vi "ASYNC_Adam_server.vi"(3 "Values":dbl[](array[numeric]) format="%.2f", 4 "Client Name":string="G3_3 HD", 5 "Channel Names":string[](array[string])) -> (0 "Scan Comments":string[](array[string]), 2 "Calibrated Units":dbl[](array[numeric]) format="%.2f")   [LabVIEW 2021]
uses:
  ADAM Client/Sub VIs/ADAM Controls/Channel_State.ctl
  ADAM Client/Sub VIs/ADAM Controls/Update_scan_value.ctl
  0eb1e5d3-c67c-5f4b-9ec6-5088df587a31.vi
  Anemometry/Anemometry Sub Vis/Globals/Preference_global.vi
panel:
  out "iteration":i32
  in  "delayBetweenADAMi/o(ms)":u32
  in  "Channel Name to Watch":string
  out "Call Chain":string[](array[string])
  # "Enter the Channel name that you want to watch"
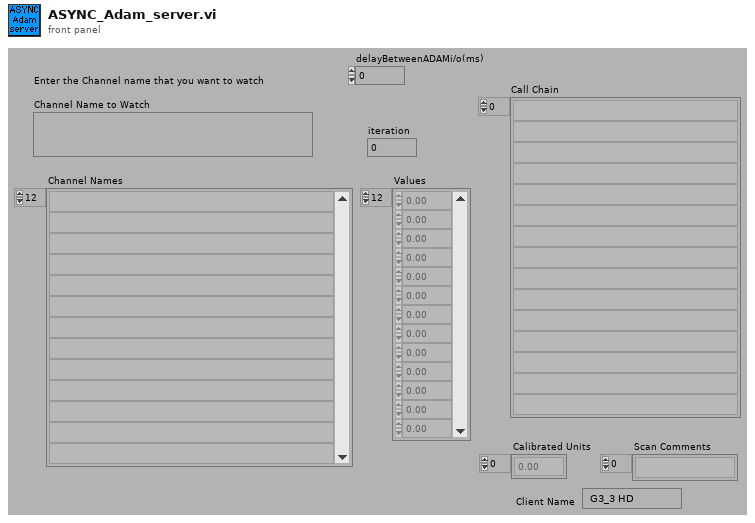
[diagram p1: front panel]
types:
  T1 = typedef "Channel_State.ctl" = enum16{"On", "Off", "Always On", "Always Off"}
  T2 = enum16{"Append to Global", "Read Global then Clear"}
  T3 = typedef "Update_scan_value.ctl" = cluster{"Channel Name":string, "New Value":dbl, "!Auto_Off":bool}
  T4 = typedef "Ch_description_ADAM.ctl" = cluster{"Ch Name":string, "Type":T5, "Function":T6, "Ch State":T1, "Calibration type":T7, "A":dbl, "B":dbl, "C":dbl, "D":dbl, "Comments":string, "Address":T8, "String":string, "Duty":u16}
  T5 = typedef "Module_type_ADAM.ctl" = string
  T6 = typedef "Function_ADAM.ctl" = enum16{"Analogue Input", "Digital Input", "Event counter", "Event rate", "Analogue Output", "Digital Output", "Relay Output"}
  T7 = typedef "Calib_type_ADAM.ctl" = string
  T8 = typedef "Address.ctl" = cluster{"Main":i32, "Ch.":i32, "Sub":i32, "Port Name":string}
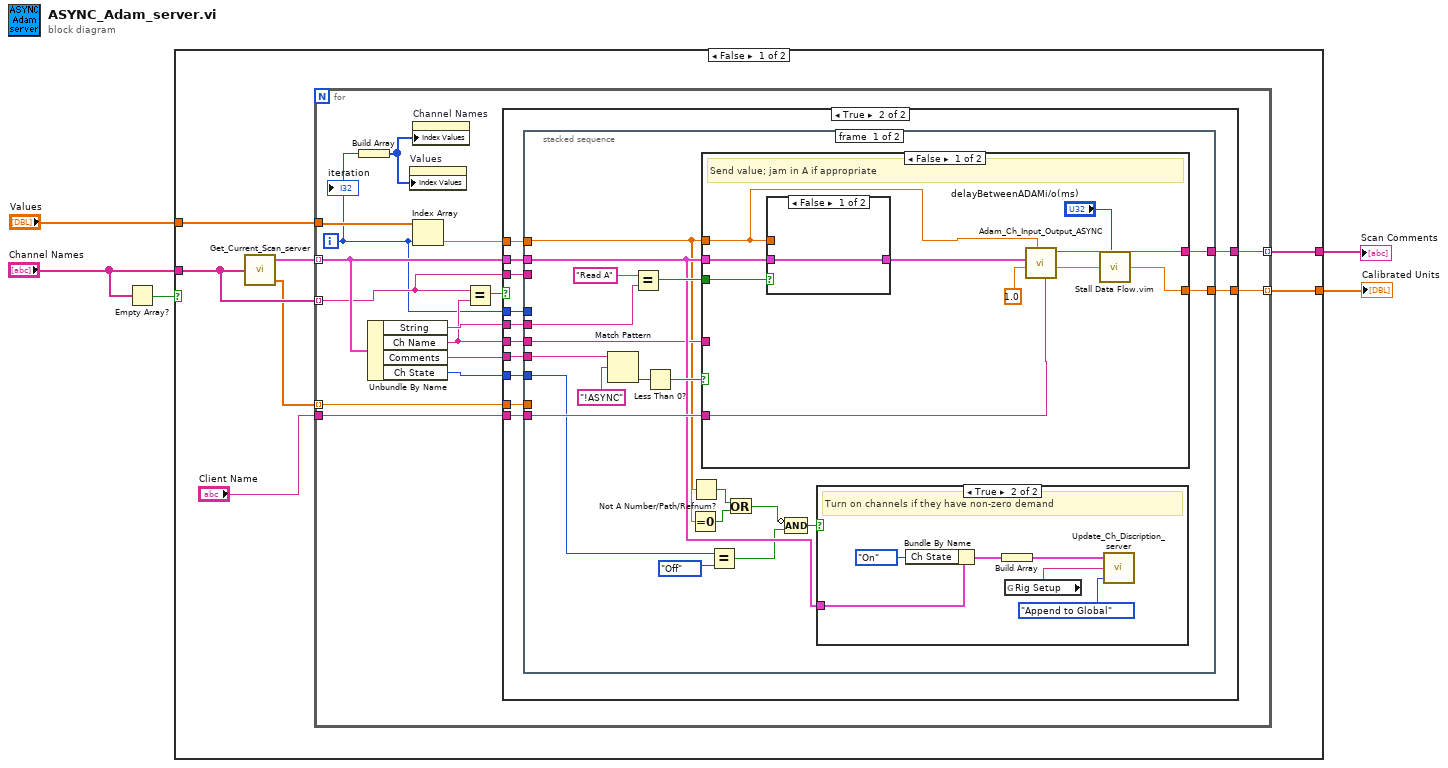
[diagram p0: block diagram]
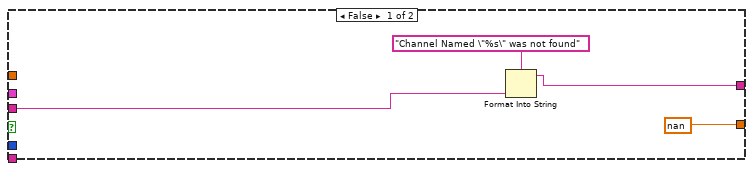
[diagram p2: hidden frame]
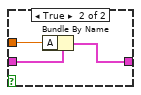
[diagram p4: hidden frame]
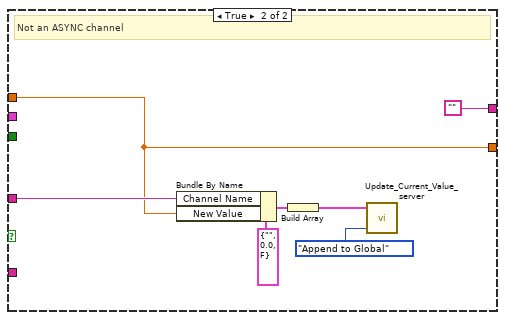
[diagram p5: hidden frame]
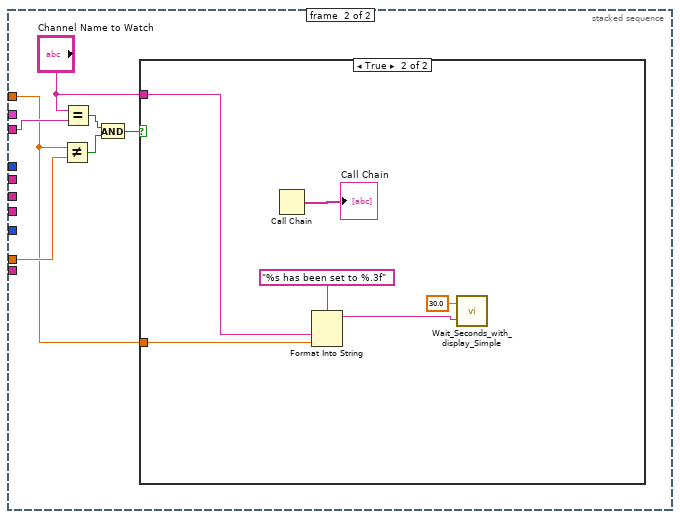
[diagram p6: hidden frame]
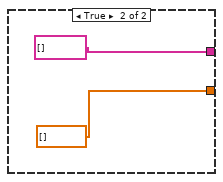
[diagram p8: hidden frame]
diagram:
  n1 = Empty Array?(array="Channel Names") -> (empty?=w3:bool)
  n2 = case shown="False" w3 {
    tunnel: "Channel Names" -> [w8 _]
    tunnel: [w10 dbl[] []] -> w5
    tunnel: [w9 string[] []] -> w4
    tunnel: "Values" -> [w7 _]
    frame False {
      n3 = call "Get_Current_Scan_server.vi"("Desired Channels"=w8) -> ("Ch Description Array"=w12:T4[], "Numerical Values"=w6:dbl[])  [unwired: 1 out]
      n4 = for {
        tunnel: w12 -> [w21] mode=indexing
        tunnel: w7 -> [w16]
        tunnel: [w27] -> w9 mode=indexing
        tunnel: [w26] -> w10 mode=indexing
        tunnel: "Client Name" -> [w25]
        tunnel: w8 -> [w17] mode=indexing
        tunnel: w6 -> [w15] mode=indexing
        i -> [w14]
        n5 = Build Array(w14) -> (w13:i32[])
        n6 = Unbundle By Name(w21) -> ("String"=w24:string, "Ch Name"=w19:string, "Comments"=w23:string, "Ch State"=w22:T1)
        n7 = property on="Values" class="Arr (strict)"("Index Values"=w13) -> ()  [unwired: 2 in, 2 out]
        n8 = property on="Channel Names" class="Arr (strict)"("Index Values"=w13) -> ()  [unwired: 2 in, 2 out]
        n9 = Index Array(array=w16, index=w14) -> (element=w20:dbl)
        n10 = Equal?(x=w17, y=w19) -> (x = y?=w18:bool)
        n11 = case shown="True" w18 {
          tunnel: [w28 w43] -> w27
          tunnel: [nan ("Calibrated units") w42] -> w26
          tunnel: w25 -> [_ w41]
          tunnel: w24 -> [_ w40]
          tunnel: w23 -> [_ w39]
          tunnel: w22 -> [_ w38]
          tunnel: w21 -> [_ w37]
          tunnel: w20 -> [_ w35]
          tunnel: w19 -> [_ w36]
          tunnel: w17 -> [w30 w34]
          tunnel: w14 -> [_ w33]
          tunnel: w15 -> [_ w32]
          frame False {
            n12 = Format Into String(format string="Channel Named \"%s\" was not found", w30) -> (resulting string=w28:string)  [unwired: 2 in, 1 out]
          }
          frame True {
            n13 = stacked-sequence {
              tunnel: [w63 _] -> w43
              tunnel: [w62 _] -> w42
              tunnel: w41 -> [w61 _]
              tunnel: w40 -> [w58 _]
              tunnel: w39 -> [w56 _]
              tunnel: w38 -> [w52 _]
              tunnel: w37 -> [w51 _]
              tunnel: w36 -> [w48 _]
              tunnel: w35 -> [w47 w91]
              tunnel: w34 -> [_ w97]
              tunnel: w33 -> [_ _]
              tunnel: w32 -> [_ w93]
              frame #0 {
                n14 = Match Pattern(string=w56, regular expression="!ASYNC" ("String to match")) -> (offset past match=w55:i32)  [unwired: 4 out]
                n15 = Equal?(x="Read A", y=w58) -> (x = y?=w60:bool)
                n16 = Less Than 0?(x=w55) -> (x < 0?=w54:bool)
                n17 = Equal To 0?(x=w47) -> (x = 0?=w46:bool)
                n18 = Not A Number/Path/Refnum?(number/path/refnum=w47) -> (NaN/Path/Refnum?=w45:bool)
                n19 = case shown="False" w54 {
                  tunnel: [w79 ""] -> w63
                  tunnel: [w71 w85] -> w62
                  tunnel: w61 -> [w77 _]
                  tunnel: w60 -> [w76 _]
                  tunnel: w51 -> [w75 _]
                  tunnel: w47 -> [w74 w85]
                  tunnel: w48 -> [_ w89]
                  frame False {
                    # "Send value; jam in A if appropriate"
                    n20 = case shown="False" w76 {
                      tunnel: w75 -> [w80 w83]
                      tunnel: w74 -> [_ w82]
                      tunnel: [w80 w81] -> w73
                      frame False {
                      }
                      frame True {
                        n21 = Bundle By Name(cluster=w83, "A"=w82) -> (w81:T4)
                      }
                    }
                    n22 = call "Adam_Ch_Input_Output_ASYNC.vi"("Client Name"=w77, "Value to Output"=w74, "Scan Period"=1.0, "Ch Description"=w73) -> ("Calibrated units"=w78:dbl, "Scan comment"=w79:string)  [unwired: 3 in, 3 out]
                    n23 = call "Stall Data Flow.vim"("value in"=w78, "milliseconds to wait"="delayBetweenADAMi/o(ms)") -> ("value out"=w71:dbl)  [unwired: 1 out]
                  }
                  frame True {
                    # "Not an ASYNC channel"
                    n24 = Bundle By Name(cluster=T3 {"Channel Name"="", "New Value"=0.0, "!Auto_Off"=FALSE} ("Update Scan Value Cluster"), "Channel Name"=w89, "New Value"=w85) -> (w88:T3)
                    n25 = Build Array(w88) -> (w87:T3[])
                    n26 = call "Update_Current_Value_server.vi"("Mode"=T2."Append to Global", "Update array in"=w87) -> ()  [unwired: 1 in, 1 out]
                  }
                }
                n27 = Equal?(x=w52, y=Channel_State."Off" ("Ch State")) -> (x = y?=w50:bool)
                n28 = Or(x=w45, y=w46) -> (x .or. y?=w44:bool)
                n29 = Compound Arithmetic op=AND(invert w44, w50) -> (w49:bool)
                n30 = case shown="True" w49 {
                  tunnel: w51 -> [_ w67]
                  frame False {
                  }
                  frame True {
                    # "Turn on channels if they have non-zero demand"
                    n31 = Bundle By Name(cluster=w67, "Ch State"=Channel_State."On") -> (w65:T4)
                    n32 = Build Array(w65) -> (w64:T4[])
                    n33 = global read "Preference_global.vi" "Rig Setup"() -> (w68:string)
                    n34 = call "Update_Ch_Discription_server.vi"("Mode"=T2."Append to Global", "Client HD name"=w68, "Channels to update In"=w64) -> ()  [unwired: 1 out]
                  }
                }
              }
              frame #1 {
                n35 = Not Equal?(x=w91, y=w93) -> (x != y?=w96:bool)
                n36 = Equal?(x="Channel Name to Watch", y=w97) -> (x = y?=w95:bool)
                n37 = And(x=w95, y=w96) -> (x .and. y?=w94:bool)
                n38 = case shown="True" w94 {
                  tunnel: "Channel Name to Watch" -> [_ w99]
                  tunnel: w91 -> [_ w98]
                  frame False {
                  }
                  frame True {
                    n39 = Call Chain() -> (call chain=→"Call Chain":string[])
                    n40 = Format Into String(format string="%s has been set to %.3f", w99, w98) -> (resulting string=w103:string)  [unwired: 2 in, 1 out]
                    n41 = call "Wait_Seconds_with_display_Simple.vi"("Message"=w103, "Seconds to wait"=30.0) -> ()  [unwired: 1 in, 1 out]
                  }
                }
              }
            }
          }
        }
        "iteration" <- w14
      }
    }
    frame True {
    }
  }
  "Calibrated Units" <- w5
  "Scan Comments" <- w4
